vi "raw_lock.vi"() -> ()   [LabVIEW 2022 SP3]
panel:
  out "error out 2":errorcluster
  out "error out":errorcluster
  in  "Tab Control":T1(tab)
  in  "ENTER PIN":string
  in  "Refresh Button 2":bool
  out "Boolean 5":bool
  out "Boolean 4":bool
  out "Boolean 3":bool
  out "Boolean 2":bool
  in  "stop":bool
  in  "comport 2":bool
  in  "comport":bool
  in  "settings":bool
  in  "tytyt":bool
  out "1":dbl format="%02d"
  in  "1 5":bool
  in  "1 4":bool
  in  "1 3":bool
  in  "1 2":bool
  in  "comport 3":bool
  in  "comport 4":bool
  in  "Cancel Button":bool
  in  "Previous Button":bool
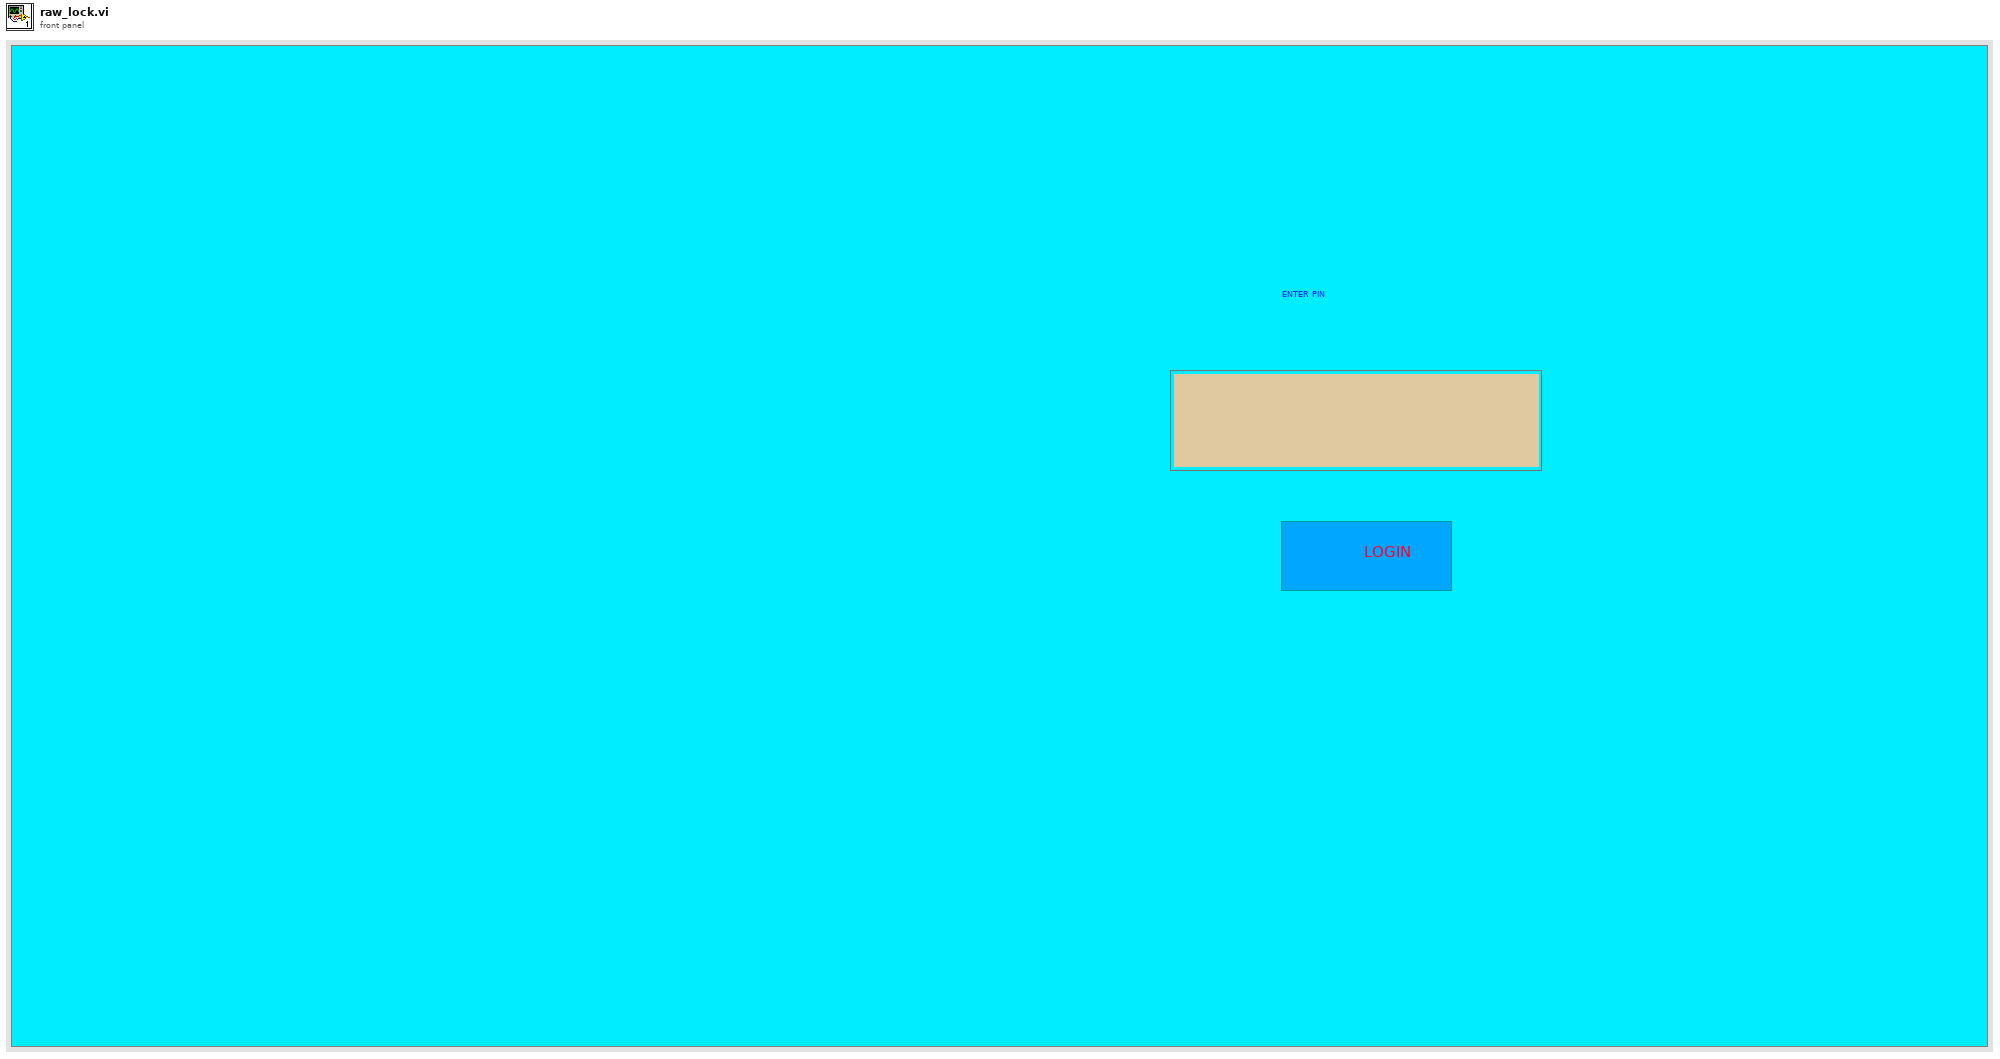
[diagram p1: front panel]
types:
  T1 = enum32{"Page 1", "Page 2", "Page 3", "Page 4", "Page 5", "Page 6"}
  T2 = enum32{"Page 1", "Page 2", "Page 3", "Page 4", "Page 5"}
  T3 = enum16{"open", "replace", "create", "open or create", "replace or create", "replace or create with confirmation"}
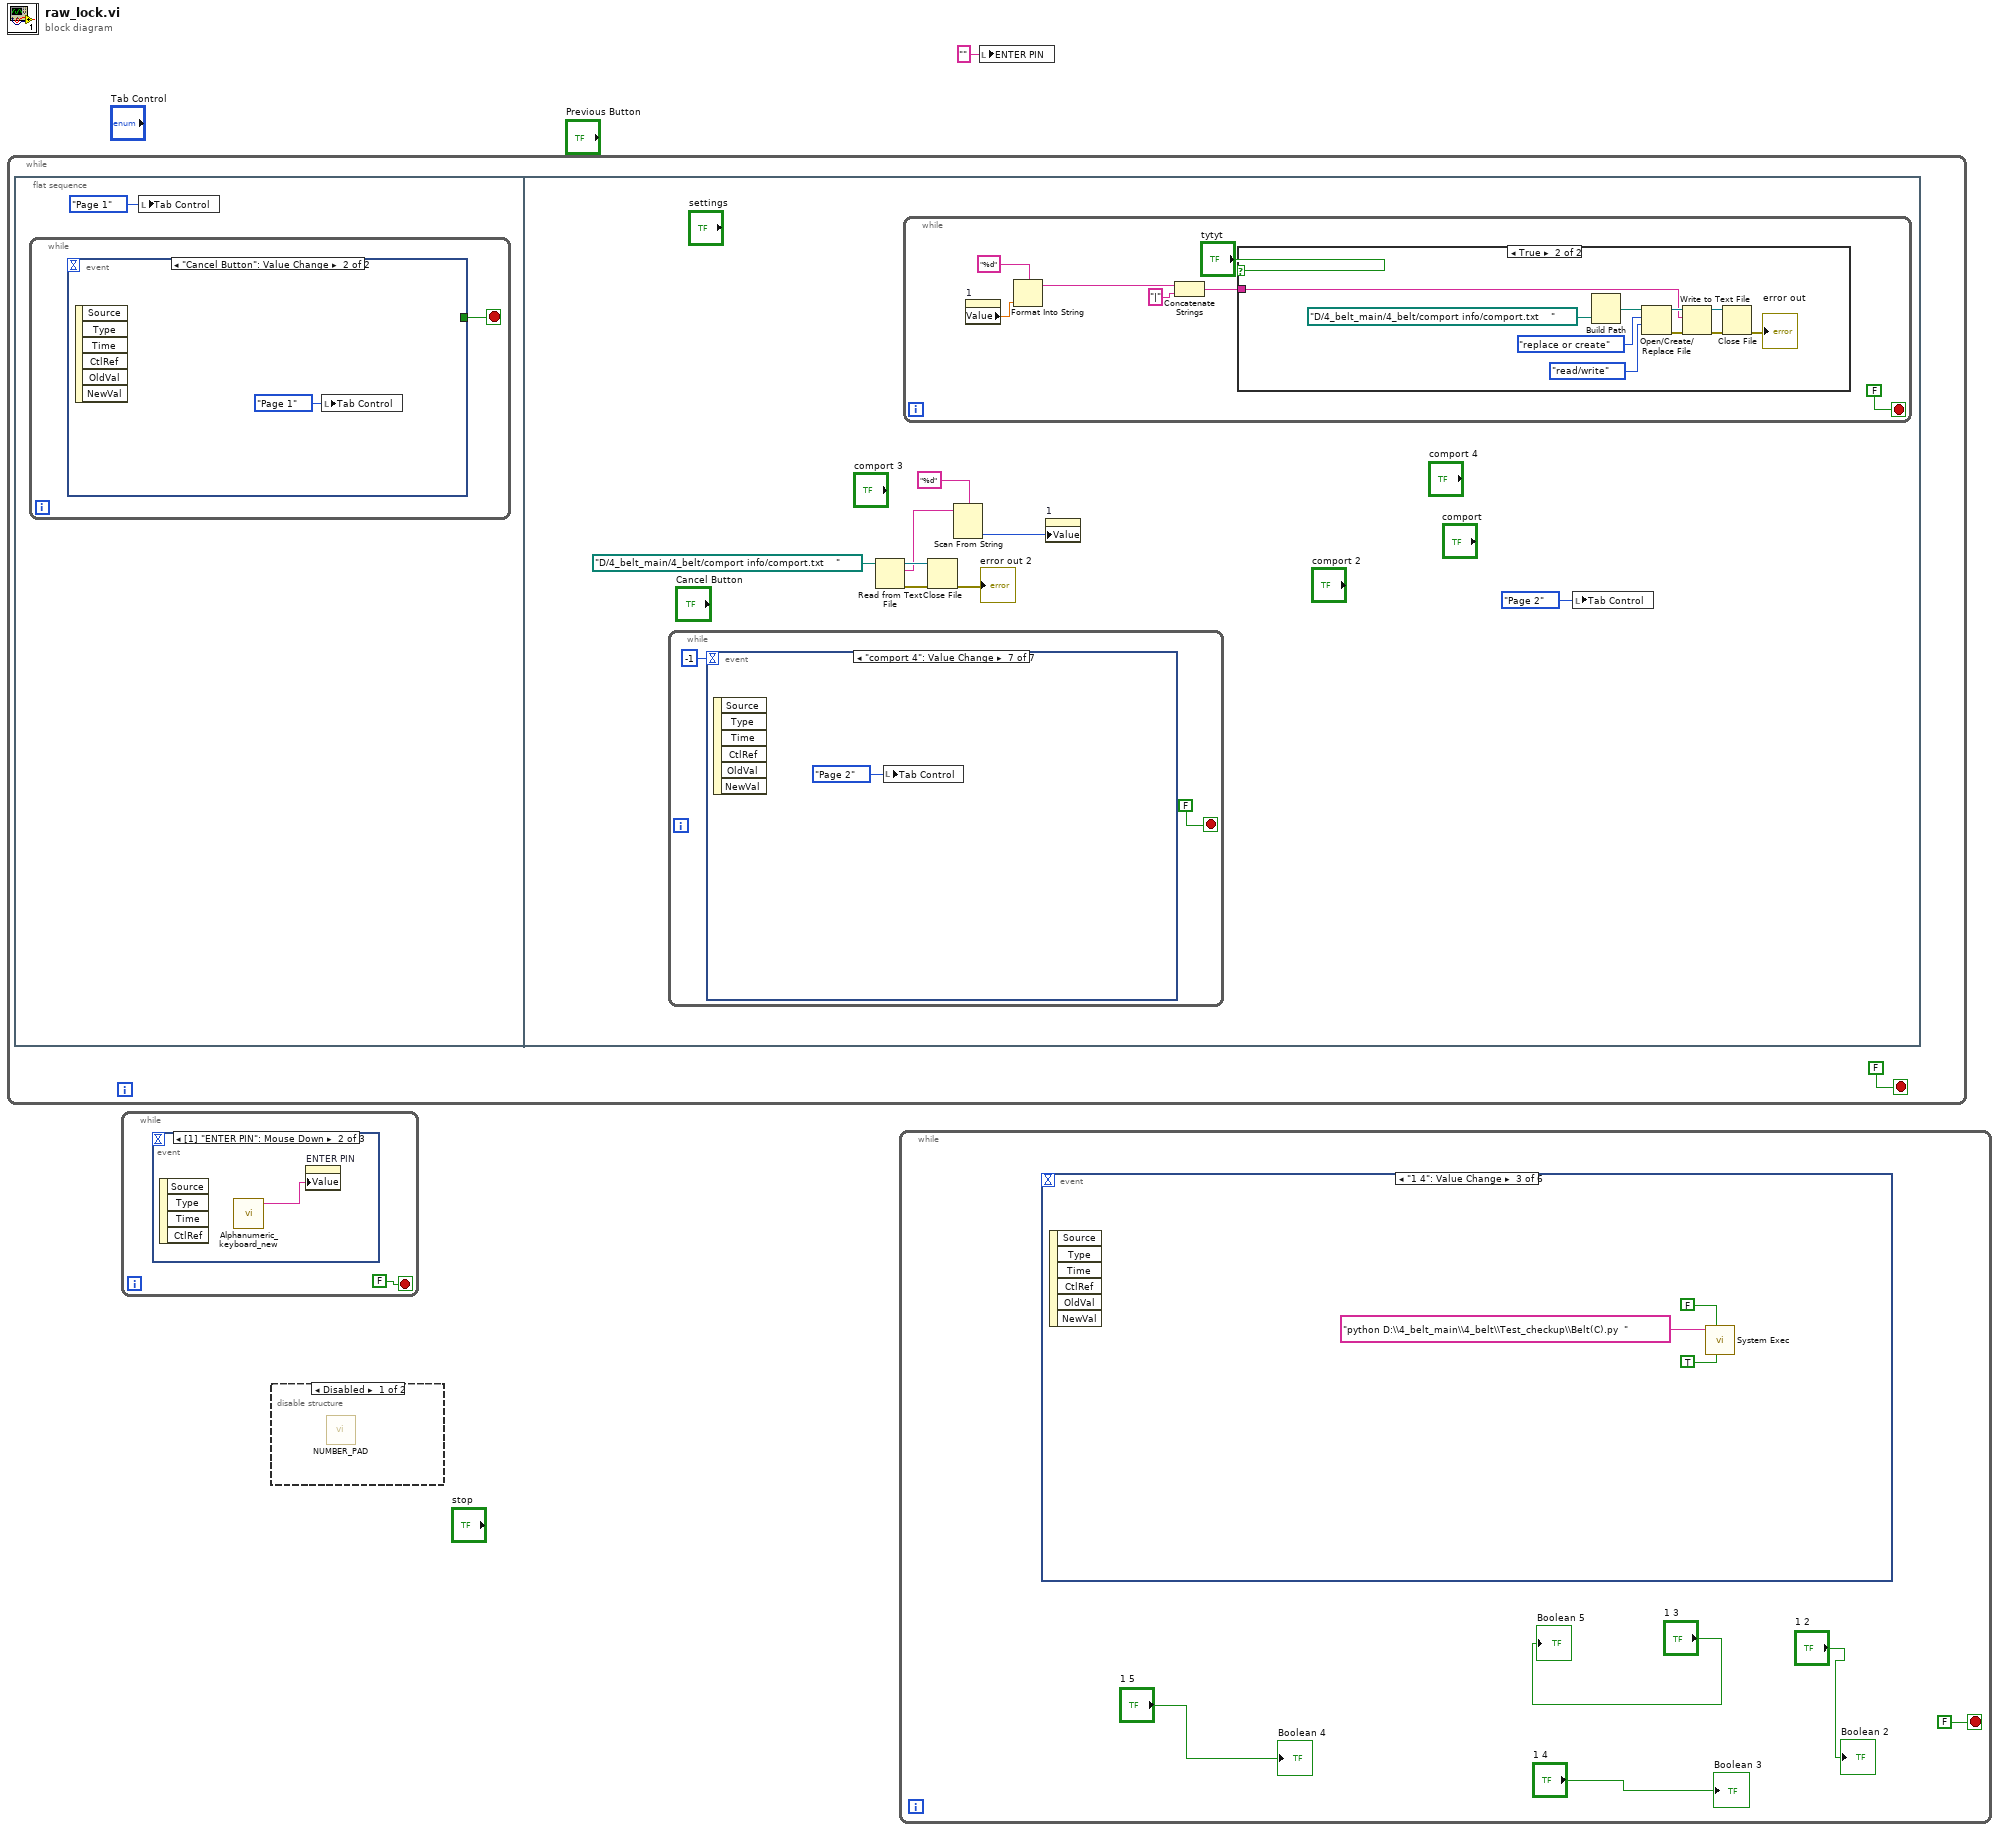
[diagram p0: block diagram]
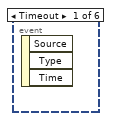
[diagram p3: hidden frame]
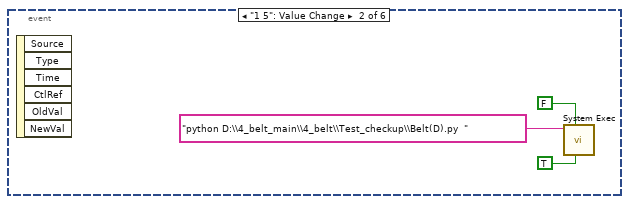
[diagram p4: hidden frame]
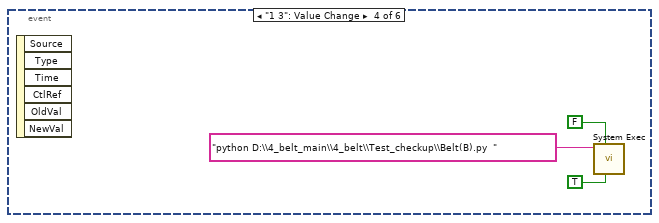
[diagram p5: hidden frame]
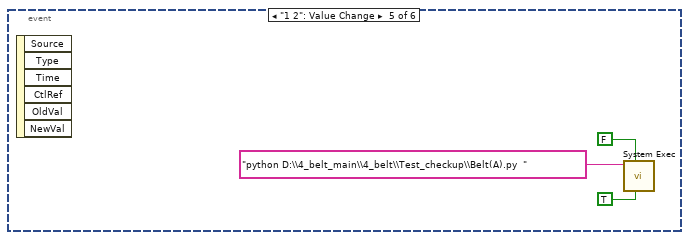
[diagram p6: hidden frame]
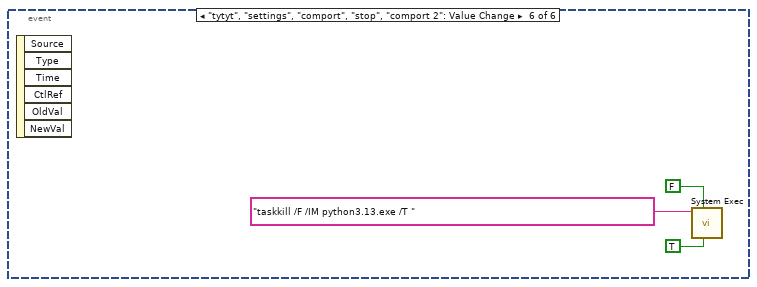
[diagram p7: hidden frame]
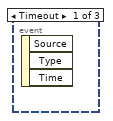
[diagram p8: hidden frame]
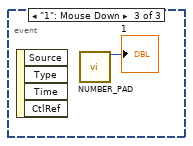
[diagram p9: hidden frame]
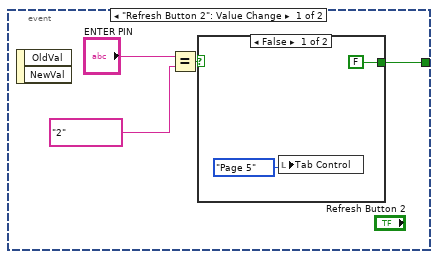
[diagram p10: hidden frame]
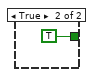
[diagram p11: hidden frame]
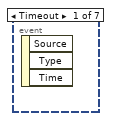
[diagram p12: hidden frame]
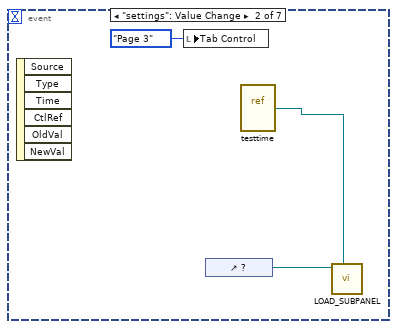
[diagram p13: hidden frame]
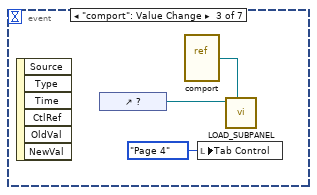
[diagram p14: hidden frame]
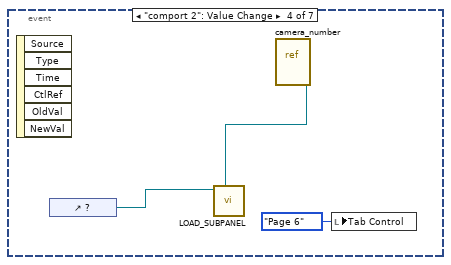
[diagram p15: hidden frame]
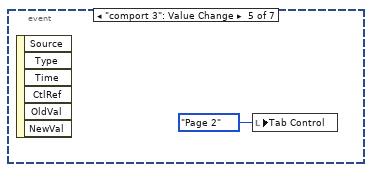
[diagram p16: hidden frame]
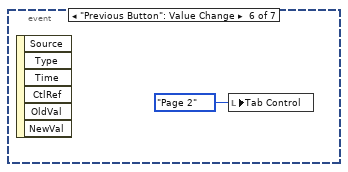
[diagram p17: hidden frame]
diagram:
  n1 = while {
    stop <- FALSE stop-if-true
    n2 = flat-sequence {
      frame #0 {
        n3 = while {
          stop <- w4 stop-if-true
          n4 = event shown="[1] \"Cancel Button\": Value Change" {
            selector: _ -> [_ _]
            dyn-events: _ -> [_ _]
            timeout: _ -> [_ _]
            tunnel: [w7 _] -> w4
            event "Refresh Button 2": Value Change {
              n5 = event-data() -> ()  [unwired: 1 in, 2 out]
              n6 = Equal?(x="ENTER PIN", y="2") -> (x = y?=w8:bool)
              n7 = case shown="False" w8 {
                tunnel: [FALSE TRUE] -> w7
                frame False {
                  n8 = local write "Tab Control"(T2."Page 5" ("Tab Control")) -> ()
                }
                frame True {
                }
              }
            }
            event "Cancel Button": Value Change {
              n9 = event-data() -> ()  [unwired: 1 in, 6 out]
              n10 = local write "Tab Control"(T2."Page 1" ("Tab Control")) -> ()
            }
          }
        }
        n11 = local write "Tab Control"(enum32{"Page 1", "Page 2"}."Page 1" ("Tab Control")) -> ()
      }
      frame #1 {
        n12 = while {
          stop <- FALSE stop-if-true
          n13 = event shown="[6] \"comport 4\": Value Change" {
            selector: _ -> [_ _ _ _ _ _ _]
            dyn-events: _ -> [_ _ _ _ _ _ _]
            timeout: -1 -> [_ _ _ _ _ _ _]
            event Timeout {
              n14 = event-data() -> ()  [unwired: 1 in, 3 out]
            }
            event "settings": Value Change {
              n15 = event-data() -> ()  [unwired: 1 in, 6 out]
              n16 = local write "Tab Control"(enum32{"Page 1", "Page 2", "Page 3"}."Page 3" ("Tab Control")) -> ()
              n17 = control-ref of="?"() -> (w24:refnum<vi>)
              n18 = vi-ref "testtime.vi"() -> (w23:refnum<vi>)
              n19 = call "LOAD_SUBPANEL.vi"("SubPanel in"=w24, "VI Ref"=w23) -> ()  [unwired: 8 in, 1 out]
            }
            event "comport": Value Change {
              n20 = event-data() -> ()  [unwired: 1 in, 6 out]
              n21 = control-ref of="?"() -> (w28:refnum<vi>)
              n22 = vi-ref "comport.vi"() -> (w27:refnum<vi>)
              n23 = local write "Tab Control"(enum32{"Page 1", "Page 2", "Page 3", "Page 4"}."Page 4" ("Tab Control")) -> ()
              n24 = call "LOAD_SUBPANEL.vi"("SubPanel in"=w28, "VI Ref"=w27) -> ()  [unwired: 8 in, 1 out]
            }
            event "comport 2": Value Change {
              n25 = event-data() -> ()  [unwired: 1 in, 6 out]
              n26 = control-ref of="?"() -> (w29:refnum<vi>)
              n27 = vi-ref "camera_number.vi"() -> (w31:refnum<vi>)
              n28 = call "LOAD_SUBPANEL.vi"("SubPanel in"=w29, "VI Ref"=w31) -> ()  [unwired: 8 in, 1 out]
              n29 = local write "Tab Control"(T1."Page 6" ("Tab Control")) -> ()
            }
            event "comport 3": Value Change {
              n30 = event-data() -> ()  [unwired: 1 in, 6 out]
              n31 = local write "Tab Control"(enum32{"Page 1", "Page 2"}."Page 2" ("Tab Control")) -> ()
            }
            event "Previous Button": Value Change {
              n32 = event-data() -> ()  [unwired: 1 in, 6 out]
              n33 = local write "Tab Control"(enum32{"Page 1", "Page 2"}."Page 2" ("Tab Control")) -> ()
            }
            event "comport 4": Value Change {
              n34 = event-data() -> ()  [unwired: 1 in, 6 out]
              n35 = local write "Tab Control"(enum32{"Page 1", "Page 2"}."Page 2" ("Tab Control")) -> ()
            }
          }
        }
        n36 = Read from Text File(file (use dialog)=path "D:/4_belt_main/4_belt/comport info/comport.txt    " ("name or relative path")) -> (refnum out=w20:refnum<file>, text=w17:string, error out=w19:errorcluster)  [unwired: 3 in, 1 out]
        n37 = while {
          stop <- FALSE stop-if-true
          n38 = property on="1" class="DigNum (strict)"() -> ("Value"=w36:dbl)  [unwired: 2 in, 2 out]
          n39 = Format Into String "Format Into String"(format string="%d" ("resulting string"), w36) -> (resulting string=w40:string)  [unwired: 2 in, 1 out]
          n40 = Concatenate Strings(w40, "|" ("string")) -> (w41:string)
          n41 = case shown="True" "tytyt" {
            tunnel: w41 -> [_ w43]
            frame False {
            }
            frame True {
              n42 = Build Path(name or relative path=path "D:/4_belt_main/4_belt/comport info/comport.txt    ") -> (appended path=w51:path)  [unwired: 1 in]
              n43 = Open/Create/Replace File(file path (use dialog)=w51, operation (0:open)=T3."replace or create", access (0:read/write)=enum16{"read/write", "read-only", "write-only"}."read/write") -> (refnum out=w48:refnum<file>, error out=w47:errorcluster)  [unwired: 3 in, 1 out]
              n44 = Write to Text File(file (use dialog)=w48, text=w43, error in=w47) -> (refnum out=w46:refnum<file>, error out=w45:errorcluster)  [unwired: 1 in, 1 out]
              n45 = Close File(refnum=w46, error in=w45) -> (error out=→"error out":errorcluster)  [unwired: 1 out]
            }
          }
        }
        n46 = Close File(refnum=w20, error in=w19) -> (error out=→"error out 2":errorcluster)  [unwired: 1 out]
        n47 = Scan From String(format string="%d", input string=w17) -> (output 1=w16:i32)  [unwired: 3 in, 3 out]
        n48 = property on="1" class="DigNum (strict)"("Value"=w16) -> ()  [unwired: 2 in, 2 out]
        n49 = local write "Tab Control"(enum32{"Page 1", "Page 2"}."Page 2" ("Tab Control")) -> ()
      }
    }
  }
  n50 = while {
    stop <- FALSE stop-if-true
    n51 = event shown="[1] \"ENTER PIN\": Mouse Down" {
      selector: _ -> [_ _ _]
      dyn-events: _ -> [_ _ _]
      timeout: _ -> [_ _ _]
      event Timeout {
        n52 = event-data() -> ()  [unwired: 1 in, 3 out]
      }
      event "ENTER PIN": Mouse Down {
        n53 = event-data() -> ()  [unwired: 1 in, 4 out]
        n54 = call "Alphanumeric_keyboard_new.vi"() -> ("New String"=w53:string)  [unwired: 2 in, 2 out]
        n55 = property on="ENTER PIN" class="Str"("Value"=w53) -> ()  [unwired: 2 in, 2 out]
      }
      event "1": Mouse Down {
        n56 = event-data() -> ()  [unwired: 1 in, 4 out]
        n57 = call "NUMBER_PAD.vi"() -> ("number (out)"=→"1":i32)  [unwired: 15 in]
      }
    }
  }
  n58 = disable-structure shown="Disabled" {
    frame Disabled {
      n59 = call "NUMBER_PAD.vi"() -> ()  [unwired: 15 in, 1 out]
    }
    frame Enabled {
    }
  }
  n60 = while {
    stop <- FALSE stop-if-true
    n61 = event shown="[2] \"1 4\": Value Change" {
      selector: _ -> [_ _ _ _ _ _]
      dyn-events: _ -> [_ _ _ _ _ _]
      timeout: _ -> [_ _ _ _ _ _]
      event Timeout {
        n62 = event-data() -> ()  [unwired: 1 in, 3 out]
      }
      event "1 5": Value Change {
        n63 = event-data() -> ()  [unwired: 1 in, 6 out]
        n64 = call <vilib>:"System Exec.vi"("run minimized? (F)"=TRUE, "wait until completion? (T)"=FALSE, "command line"="python D:\\4_belt_main\\4_belt\\Test_checkup\\Belt(D).py  ") -> ()  [unwired: 5 in, 4 out]
      }
      event "1 4": Value Change {
        n65 = event-data() -> ()  [unwired: 1 in, 6 out]
        n66 = call <vilib>:"System Exec.vi"("run minimized? (F)"=TRUE, "wait until completion? (T)"=FALSE, "command line"="python D:\\4_belt_main\\4_belt\\Test_checkup\\Belt(C).py  ") -> ()  [unwired: 5 in, 4 out]
      }
      event "1 3": Value Change {
        n67 = event-data() -> ()  [unwired: 1 in, 6 out]
        n68 = call <vilib>:"System Exec.vi"("run minimized? (F)"=TRUE, "wait until completion? (T)"=FALSE, "command line"="python D:\\4_belt_main\\4_belt\\Test_checkup\\Belt(B).py  ") -> ()  [unwired: 5 in, 4 out]
      }
      event "1 2": Value Change {
        n69 = event-data() -> ()  [unwired: 1 in, 6 out]
        n70 = call <vilib>:"System Exec.vi"("run minimized? (F)"=TRUE, "wait until completion? (T)"=FALSE, "command line"="python D:\\4_belt_main\\4_belt\\Test_checkup\\Belt(A).py  ") -> ()  [unwired: 5 in, 4 out]
      }
      event "tytyt", "settings", "comport", "stop", "comport 2": Value Change {
        n71 = event-data() -> ()  [unwired: 1 in, 6 out]
        n72 = call <vilib>:"System Exec.vi"("run minimized? (F)"=TRUE, "wait until completion? (T)"=FALSE, "command line"="taskkill /F /IM python3.13.exe /T ") -> ()  [unwired: 5 in, 4 out]
      }
    }
    "Boolean 2" <- "1 2"
    "Boolean 3" <- "1 4"
    "Boolean 5" <- "1 3"
    "Boolean 4" <- "1 5"
  }
  n73 = local write "ENTER PIN"("" ("ENTER PIN")) -> ()
